vi "3.4.vi"() -> ()   [LabVIEW 2017]
panel:
  in  "字符串 2":string
  in  "字符串":string
  out "长度":i32
  out "结果字符串":string
  in  "输入 2":dbl
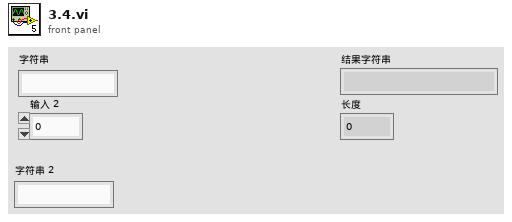
[diagram p1: front panel]
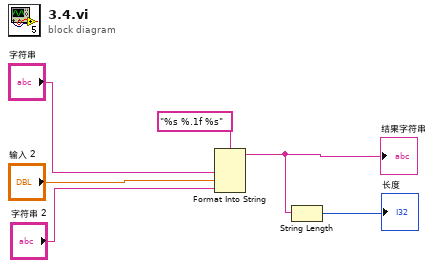
[diagram p0: block diagram]
diagram:
  n1 = Format Into String(format string="%s %.1f %s" ("格式字符串"), "字符串", "输入 2", "字符串 2") -> (resulting string=w5:string)  [unwired: 2 in, 1 out]
  "结果字符串" <- w5
  n2 = String Length(string=w5) -> (length=→"长度":i32)
